vi "reset sesion.vi"(8 "error in (no error)":errorcluster, 11 "5785_3.2GHz_one channel in":refnum<class "5785_3.2GHz_one channel.lvclass">) -> (0 "error out":errorcluster, 3 "5785_3.2GHz_one channel out":refnum<class "5785_3.2GHz_one channel.lvclass">)   [LabVIEW 2021, in "5785_3.2GHz_one channel.lvclass"]
uses:
  5785_3.2GHz_one channel.lvclass
  5785_3.2GHz_one channel.lvclass/5785_3.2GHz_one channel.ctl
  <vilib>/rvi/interface/nirviReadWriteControl/nirviReadWriteControl.xnode
  <instrlib>/_niInstr/Streaming/v1/Host/niInstr Streaming v1 Host.lvlib
  NiFpgaLv.dll
  <vilib>/Utility/error.llb/Error Cluster From Error Code.vi
  <vilib>/rvi/interface/Simulation/niFpgaSimulationCallBeginRW.vi
  <vilib>/rvi/errors/niLvFpgaAdjustHostInterfaceError.vi
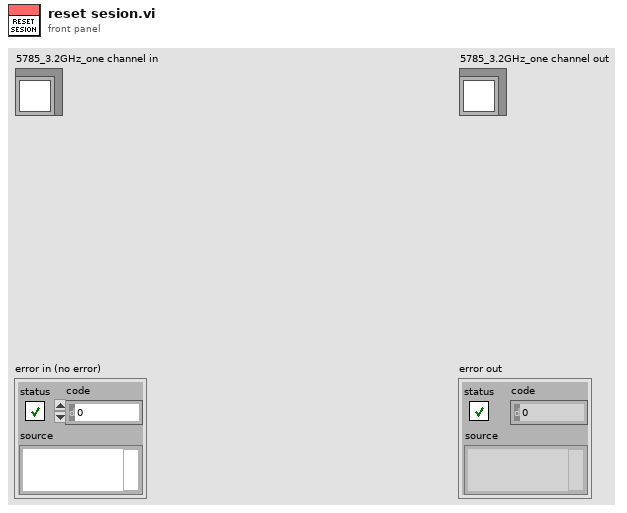
[diagram p1: front panel]
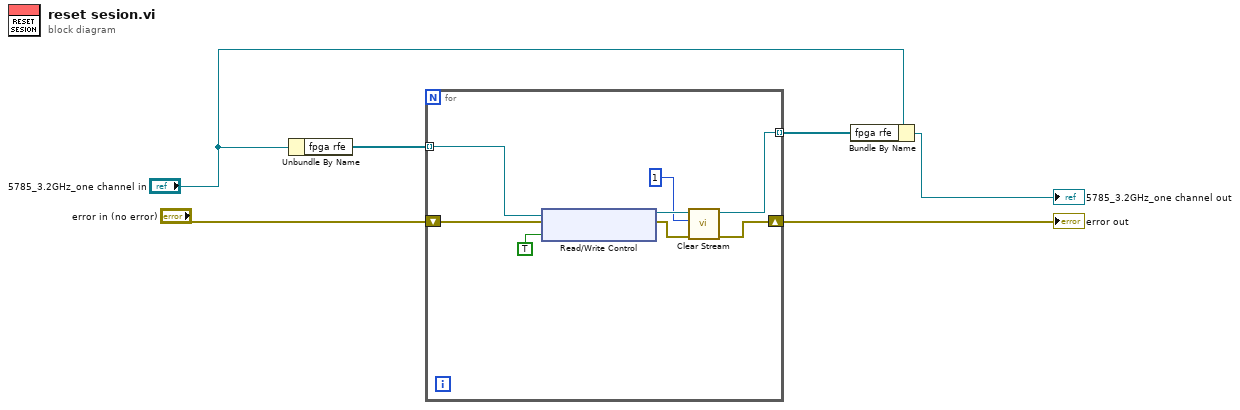
[diagram p0: block diagram]
diagram:
  n1 = Unbundle By Name("5785_3.2GHz_one channel in") -> ("fpga rfe"=w6:refnum<k20>[])
  n2 = for {
    tunnel: w6 -> [w13] mode=indexing
    shift-right: [w8] -> w2
    shift-left: "error in (no error)" -> [w10]
    tunnel: [w7] -> w3 mode=indexing
    n3 = xnode "Read/Write Control"("FPGA VI Reference In"=w13, "error in"=w10, "reset system clock"=TRUE) -> ("FPGA VI Reference Out"=w12:refnum<k20>, "error out"=w9:errorcluster)
    n4 = call <instrlib>:"Clear Stream.vi"("error in (no error)"=w9, "stream index"=1, "refnum in"=w12) -> ("error out"=w8:errorcluster, "refnum out"=w7:refnum<k20>)  [unwired: 7 in]
  }
  "error out" <- w2
  n5 = Bundle By Name(cluster="5785_3.2GHz_one channel in", "fpga rfe"=w3) -> (→"5785_3.2GHz_one channel out":refnum<class "5785_3.2GHz_one channel.lvclass">)
